vi "Main.vi"() -> ()   [LabVIEW 2021]
doc: "This software acquires data from an NI DAQ Device, displays it, and performs analysis of the data."
uses:
  controls/File Type.ctl
  controls/Data.ctl
  controls/Configuration Settings.ctl
  controls/State.ctl
panel:
  in  "Open File Location?":bool
  in  "File Type":T1
  out "Data":dbl[][](graph)
  out "Actual Sample Rate (Hz)":dbl
  in  "Copy Graph Data":bool
  in  "Copy Graph Image":bool
  in  "Reset Settings":bool
  in  "Clear Graph":bool
  in  "Read Data File":bool
  in  "Save to File":bool
  in  "Analyse Data":bool
  in  "Acquire Data":bool
  in  "Configure Data":bool
  out "Current State":string
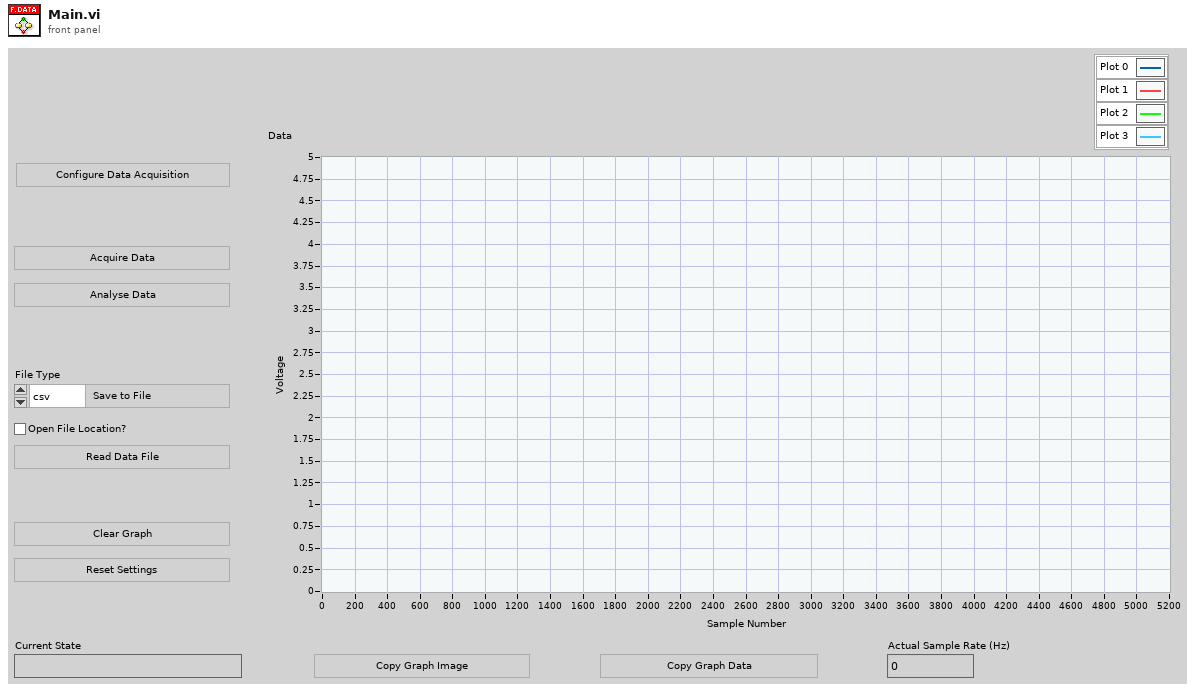
[diagram p1: front panel]
types:
  T1 = typedef "File Type.ctl" = enum16{"csv", "txt", "tdms"}
  T2 = typedef "State.ctl" = enum16{"Initialise", "Update User Interface", "Wait for Event", "Configure Data", "Acquire Data", "Reset Config Data", "Clear Data", "Analyse Data", "Save Data", "Open Data", "Error", "Stop"}
  T3 = typedef "Data.ctl" = cluster{"Configuration Settings":T4, "Data":dbl[][], "Actual Sample Rate (Hz)":dbl}
  T4 = typedef "Configuration Settings.ctl" = cluster{"Number of Samples":i32, "Desired Sample Rate (Hz)":dbl, "Minimum Value":dbl, "Maximum Value":dbl, "Physical Channels":tag}
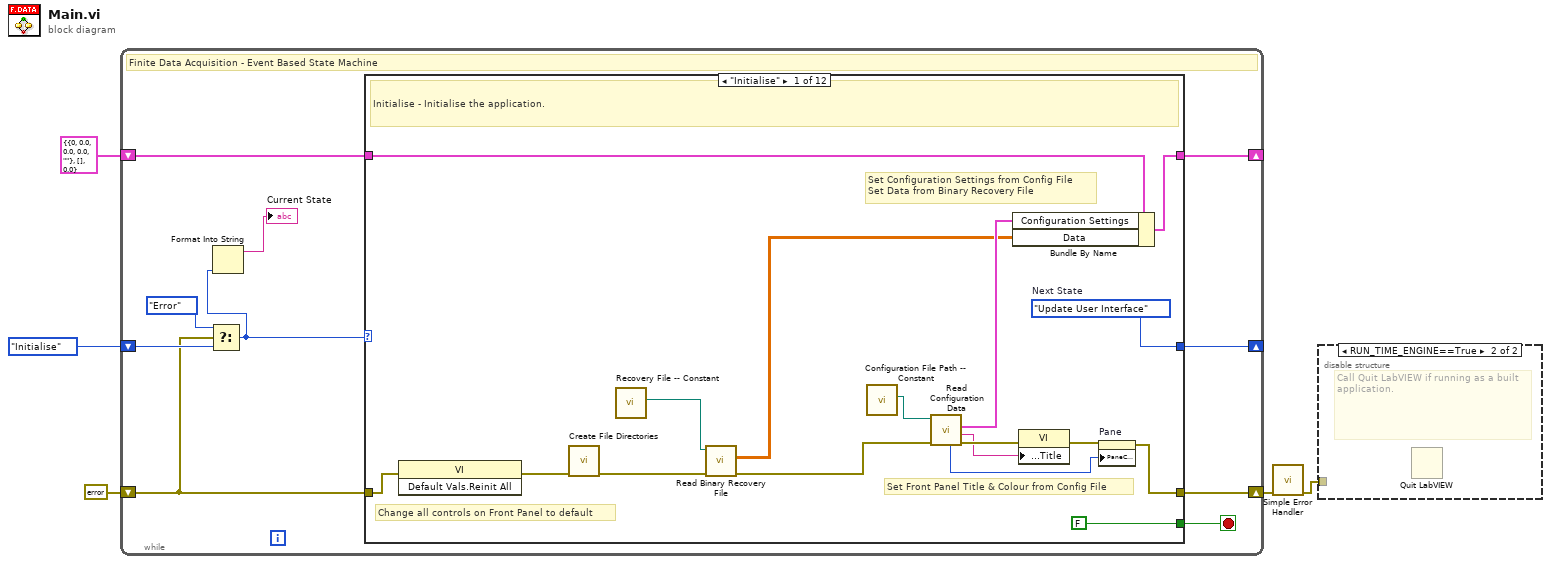
[diagram p0: block diagram]
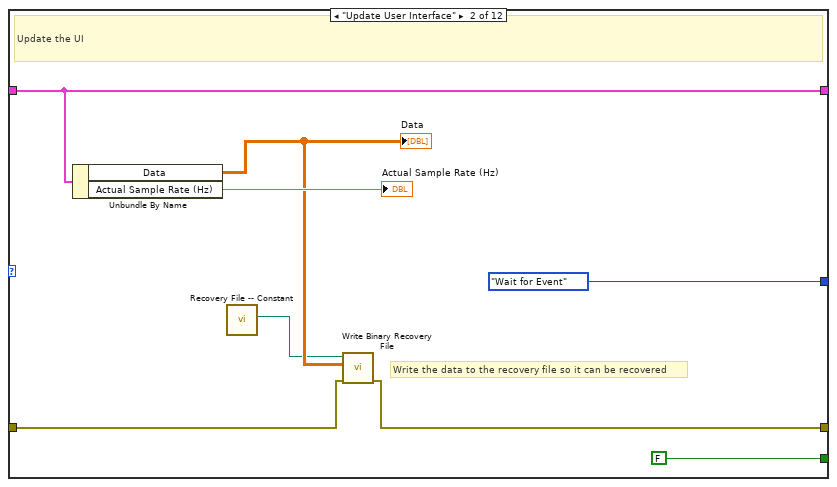
[diagram p3: hidden frame]
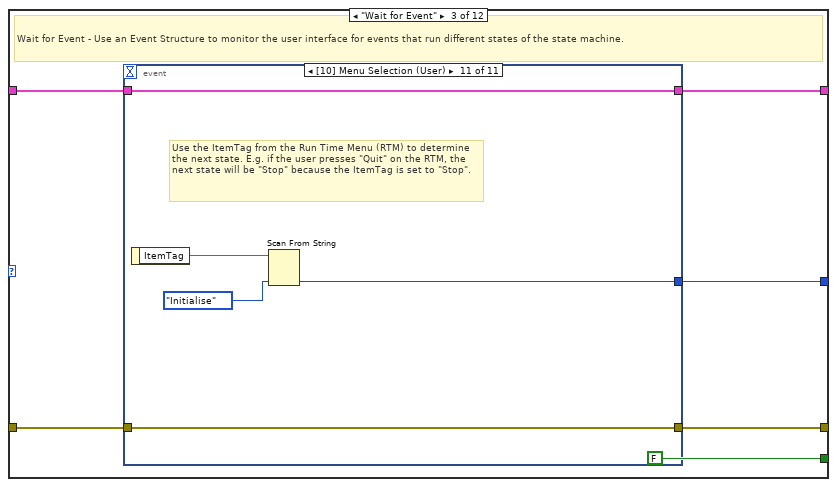
[diagram p4: hidden frame]
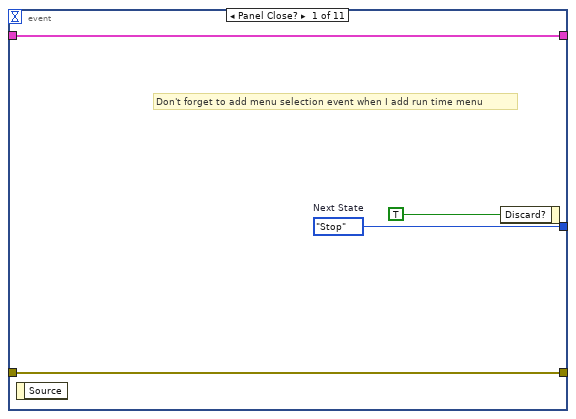
[diagram p5: hidden frame]
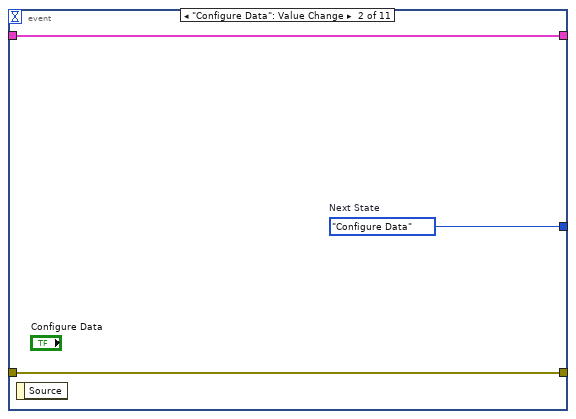
[diagram p6: hidden frame]
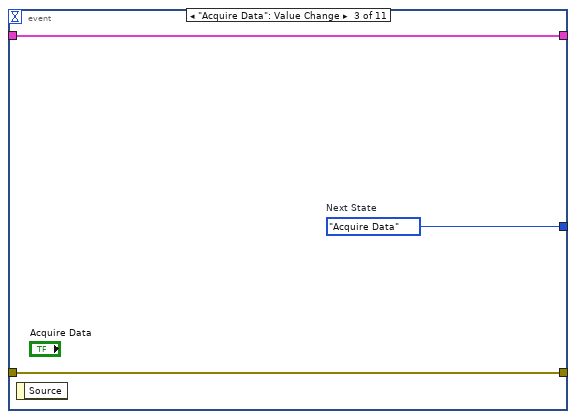
[diagram p7: hidden frame]
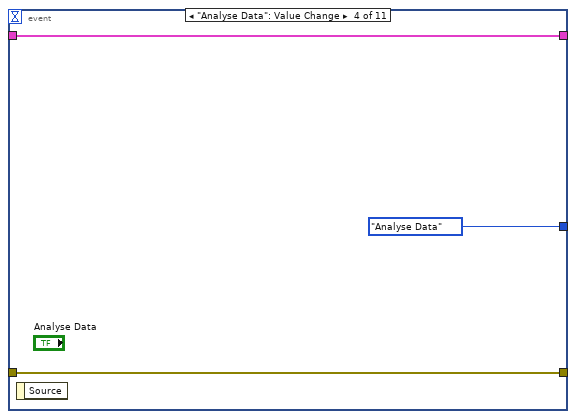
[diagram p8: hidden frame]
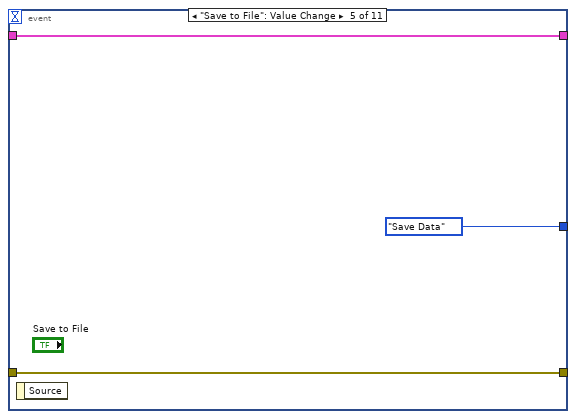
[diagram p9: hidden frame]
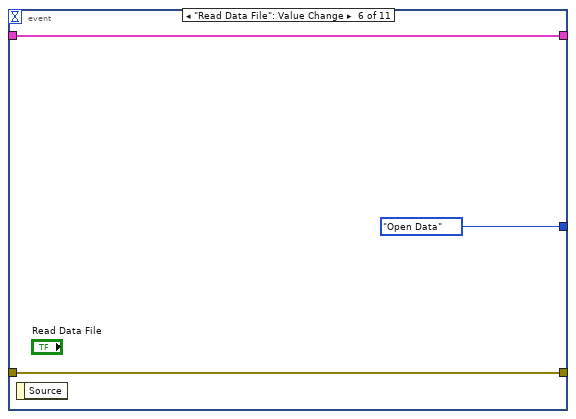
[diagram p10: hidden frame]
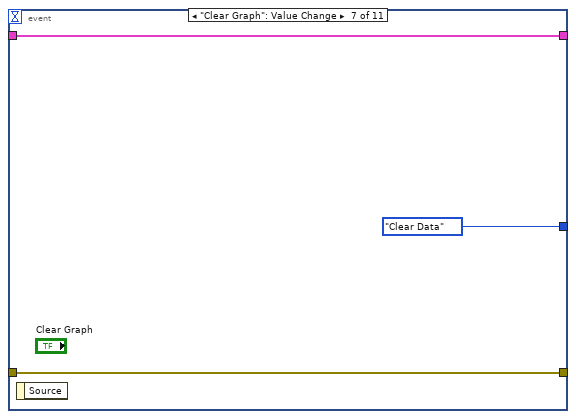
[diagram p11: hidden frame]
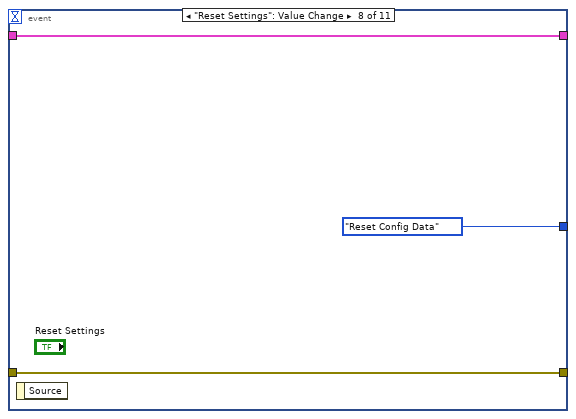
[diagram p12: hidden frame]
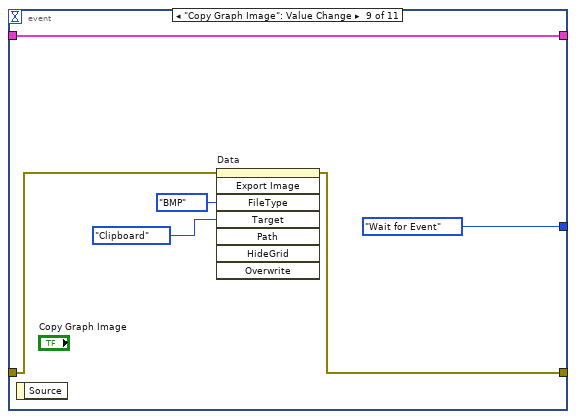
[diagram p13: hidden frame]
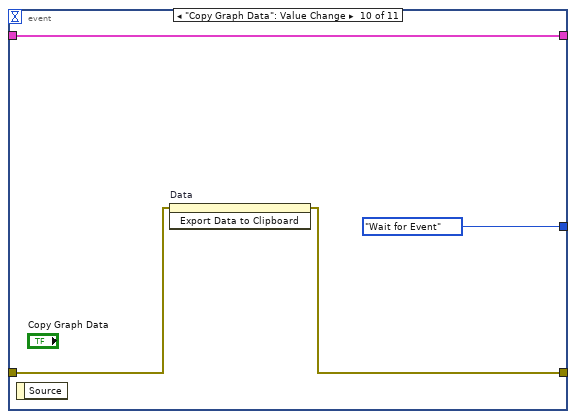
[diagram p14: hidden frame]
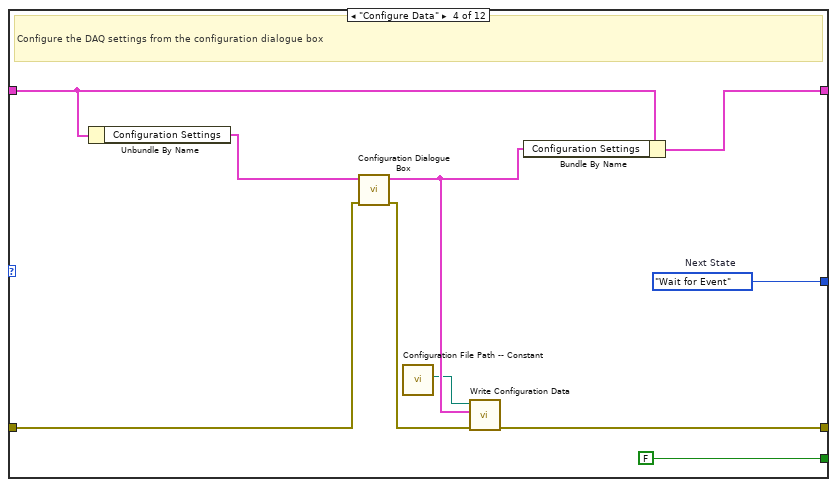
[diagram p15: hidden frame]
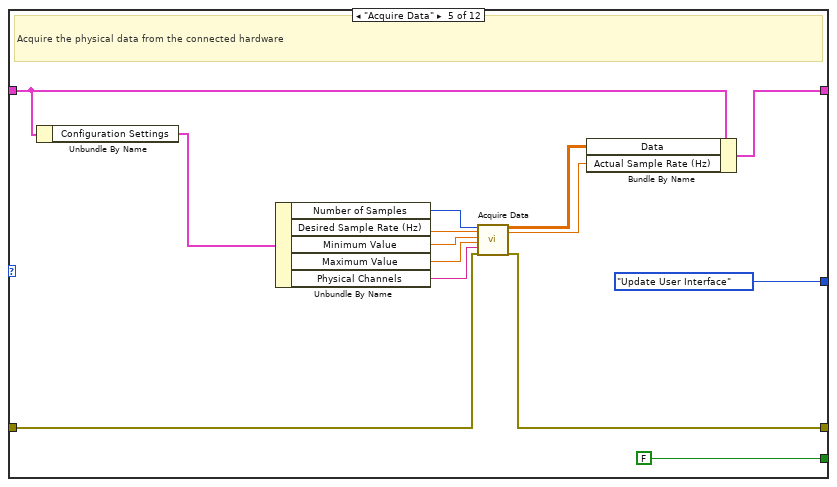
[diagram p16: hidden frame]
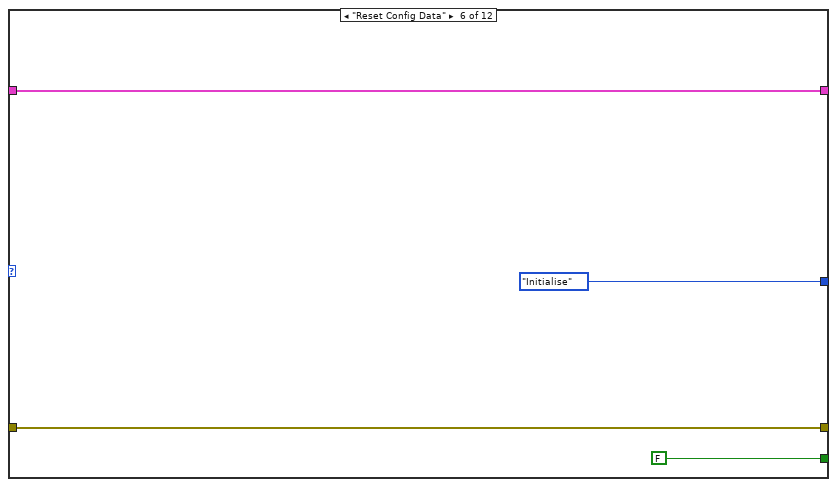
[diagram p17: hidden frame]
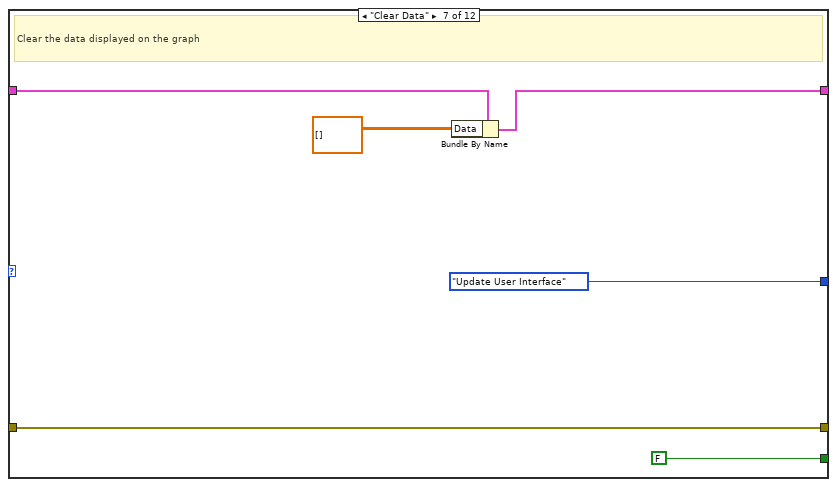
[diagram p18: hidden frame]
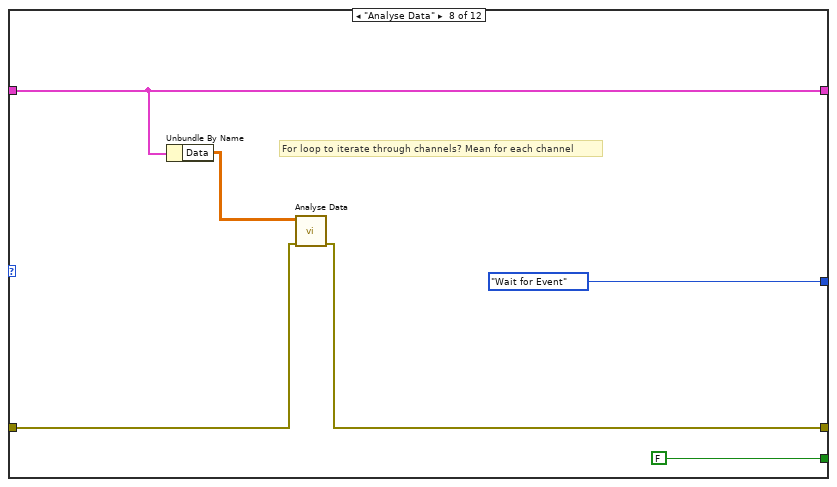
[diagram p19: hidden frame]
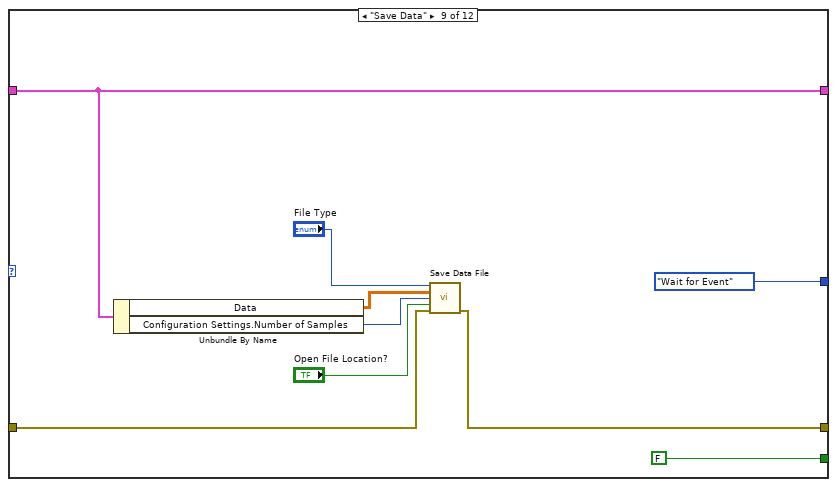
[diagram p20: hidden frame]
diagram:
  n1 = while {
    shift-right: [w15] -> _
    shift-left: State."Initialise" ("States") -> [w11]
    shift-right: [w13] -> _
    shift-left: T3 {"Configuration Settings"={"Number of Samples"=0, "Desired Sample Rate (Hz)"=0.0, "Minimum Value"=0.0, "Maximum Value"=0.0, "Physical Channels"=""}, "Data"=[], "Actual Sample Rate (Hz)"=0.0} ("Data") -> [w14]
    shift-right: [w12] -> w3
    shift-left: errorcluster {"status"=FALSE, "code"=0, "source"=""} ("error constant") -> [w9]
    stop <- w6 stop-if-true
    # "Finite Data Acquisition - Event Based State Machine"
    n2 = Select(t=State."Error", s=w9, f=w11) -> (s? t:f=w8:T2)
    n3 = Format Into String(w8) -> (resulting string=→"Current State":string)  [unwired: 3 in, 1 out]
    n4 = case shown="\"Initialise\"" w8 {
      tunnel: [w32 State."Wait for Event" ("(Value Not Used)") w46 w96 State."Update User Interface" State."Initialise" State."Update User Interface" State."Wait for Event" State."Wait for Event" w137 State."Stop" _] -> w15
      tunnel: [FALSE ("Stop Loop?") FALSE ("Stop Loop?") FALSE ("Stop Loop?") FALSE ("Stop Loop?") FALSE ("Stop Loop?") FALSE ("Stop Loop?") FALSE ("Stop Loop?") FALSE ("Stop Loop?") FALSE ("Stop Loop?") FALSE ("Stop Loop?") _ TRUE ("Stop Loop?")] -> w6
      tunnel: w14 -> [w30 w38 w44 w92 w100 w114 w117 w124 w133 w139 w191 w194]
      tunnel: [w29 w38 w43 w91 w99 w114 w116 w124 w133 w138 w191 w194] -> w13
      tunnel: w9 -> [w21 w34 w42 w93 w102 w113 w120 w122 w131 w143 w188 w193]
      tunnel: [w22 w33 w41 w87 w101 w113 w120 w121 w130 w136 errorcluster {"status"=FALSE, "code"=0, "source"=""} ("error in (no error)") w193] -> w12
      frame "Initialise" {
        w32 = State."Update User Interface"  # Next State
        # "Change all controls on Front Panel to default"
        # "Set Configuration Settings from Config File\nSet Data from Binary Recovery File"
        # "Set Front Panel Title & Colour from Config File"
        # "Initialise - Initialise the application."
        n5 = invoke class="VI" method="Default Vals.Reinit All"(error in=w21) -> (error out=w16:errorcluster)  [unwired: 2 in, 2 out]
        n6 = call "Create File Directories.vi"("error in"=w16) -> ("error out"=w20:errorcluster)  [unwired: 10 in]
        n7 = call "Recovery File -- Constant.vi"() -> ("Recovery File Path"=w19:path)  [unwired: 11 in]
        n8 = call "Read Binary Recovery File.vi"("error in"=w20, "File Path"=w19) -> ("error out"=w17:errorcluster, "Data Out"=w18:dbl[][])  [unwired: 8 in]
        n9 = call "Configuration File Path -- Constant.vi"() -> ("Configuration File Path"=w27:path)  [unwired: 11 in]
        n10 = call "Read Configuration Data.vi"("error in"=w17, "File Path"=w27) -> ("error out"=w26:errorcluster, "VI Title"=w25:string, "Configuration Settings"=w28:T4, "Panel Colour"=w24:u32)  [unwired: 6 in]
        n11 = Bundle By Name(cluster=w30, "Configuration Settings"=w28, "Data"=w18) -> (w29:T3)
        n12 = property class="VI"(error in=w26, "Front Panel.Title"=w25) -> (error out=w23:errorcluster)  [unwired: 1 in, 1 out]
        n13 = property on="Pane" class="Pane"(error in=w23, "PaneColor"=w24) -> (error out=w22:errorcluster)  [unwired: 1 in, 1 out]
      }
      frame "Update User Interface" {
        # "Write the data to the recovery file so it can be recovered"
        # "Update the UI"
        n14 = Unbundle By Name(w38) -> ("Data"=w36:dbl[][], "Actual Sample Rate (Hz)"=→"Actual Sample Rate (Hz)":dbl)
        "Data" <- w36
        n15 = call "Recovery File -- Constant.vi"() -> ("Recovery File Path"=w35:path)  [unwired: 11 in]
        n16 = call "Write Binary Recovery File.vi"("error in"=w34, "Data In"=w36, "File Path"=w35) -> ("error out"=w33:errorcluster)  [unwired: 8 in]
      }
      frame "Wait for Event" {
        # "Wait for Event - Use an Event Structure to monitor the user interface for events that run different states of the state machine."
        n17 = event shown="[10] Menu Selection (User)" {
          selector: _ -> [_ _ _ _ _ _ _ _ _ _ _]
          dyn-events: _ -> [_ _ _ _ _ _ _ _ _ _ _]
          timeout: _ -> [_ _ _ _ _ _ _ _ _ _ _]
          tunnel: [w50 w53 w56 State."Analyse Data" ("Next State") State."Save Data" ("Next State") State."Open Data" ("Next State") State."Clear Data" ("Next State") State."Reset Config Data" ("Next State") State."Wait for Event" ("Next State") State."Wait for Event" ("Next State") w82] -> w46
          tunnel: w44 -> [w49 w51 w54 w59 w62 w65 w68 w71 w77 w81 w86]
          tunnel: [w49 w51 w54 w59 w62 w65 w68 w71 w77 w81 w86] -> w43
          tunnel: w42 -> [w48 w52 w55 w58 w61 w64 w67 w70 w73 w79 w85]
          tunnel: [w48 w52 w55 w58 w61 w64 w67 w70 w72 w78 w85] -> w41
          event Panel Close? {
            w50 = State."Stop"  # Next State
            # "Don't forget to add menu selection event when I add run time menu"
            n18 = event-data() -> ()  [unwired: 1 in, 1 out]
            n19 = event-data("Discard?"=TRUE) -> ()  [unwired: 1 in, 1 out]
          }
          event "Configure Data": Value Change {
            w53 = State."Configure Data"  # Next State
            n20 = event-data() -> ()  [unwired: 1 in, 1 out]
          }
          event "Acquire Data": Value Change {
            w56 = State."Acquire Data"  # Next State
            n21 = event-data() -> ()  [unwired: 1 in, 1 out]
          }
          event "Analyse Data": Value Change {
            n22 = event-data() -> ()  [unwired: 1 in, 1 out]
          }
          event "Save to File": Value Change {
            n23 = event-data() -> ()  [unwired: 1 in, 1 out]
          }
          event "Read Data File": Value Change {
            n24 = event-data() -> ()  [unwired: 1 in, 1 out]
          }
          event "Clear Graph": Value Change {
            n25 = event-data() -> ()  [unwired: 1 in, 1 out]
          }
          event "Reset Settings": Value Change {
            n26 = event-data() -> ()  [unwired: 1 in, 1 out]
          }
          event "Copy Graph Image": Value Change {
            n27 = event-data() -> ()  [unwired: 1 in, 1 out]
            n28 = invoke on="Data" class="WFGraph (strict)" method="Export Image"(error in=w73, "FileType"=enum32{"BMP", "EPS", "EMF", "PICT"}."BMP" ("File Type"), "Target"=enum32{"File", "Clipboard"}."Clipboard") -> (error out=w72:errorcluster)  [unwired: 5 in, 7 out]
          }
          event "Copy Graph Data": Value Change {
            n29 = event-data() -> ()  [unwired: 1 in, 1 out]
            n30 = invoke on="Data" class="WFGraph (strict)" method="Export Data to Clipboard"(error in=w79) -> (error out=w78:errorcluster)  [unwired: 2 in, 2 out]
          }
          event Menu Selection (User) {
            # "Use the ItemTag from the Run Time Menu (RTM) to determine the next state. E.g. if the user presses \"Quit\" on the RTM, the next state will be \"Stop\" because the ItemTag is set to \"Stop\"."
            n31 = event-data() -> ("ItemTag"=w84:string)  [unwired: 1 in]
            n32 = Scan From String "Scan From String"(input string=w84, default 1=State."Initialise" ("States")) -> (output 1=w82:T2)  [unwired: 3 in, 3 out]
          }
        }
      }
      frame "Configure Data" {
        w96 = State."Wait for Event"  # Next State
        # "Configure the DAQ settings from the configuration dialogue box"
        n33 = Unbundle By Name(w92) -> ("Configuration Settings"=w94:T4)
        n34 = call "Configuration Dialogue Box.vi"("error in"=w93, "Configuration Settings In"=w94) -> ("error out"=w88:errorcluster, "Configuration Settings Out"=w90:T4)  [unwired: 8 in]
        n35 = call "Configuration File Path -- Constant.vi"() -> ("Configuration File Path"=w89:path)  [unwired: 11 in]
        n36 = call "Write Configuration Data.vi"("error in"=w88, "Configuration Settings"=w90, "File Path"=w89) -> ("error out"=w87:errorcluster)  [unwired: 8 in]
        n37 = Bundle By Name(cluster=w92, "Configuration Settings"=w90) -> (w91:T3)
      }
      frame "Acquire Data" {
        # "Acquire the physical data from the connected hardware"
        n38 = Unbundle By Name(w100) -> ("Configuration Settings"=w109:T4)
        n39 = Unbundle By Name(w109) -> ("Number of Samples"=w107:i32, "Desired Sample Rate (Hz)"=w106:dbl, "Minimum Value"=w105:dbl, "Maximum Value"=w104:dbl, "Physical Channels"=w103:tag)
        n40 = call "Acquire Data.vi"("Number of Samples"=w107, "Desired Sample Rate (Hz)"=w106, "Minimum Value"=w105, "Maximum Value"=w104, "Physical Channels"=w103, "error in"=w102) -> ("Data Out"=w98:dbl[][], "Actual Sample Rate (Hz)"=w97:dbl, "error out"=w101:errorcluster)  [unwired: 11 in]
        n41 = Bundle By Name(cluster=w100, "Data"=w98, "Actual Sample Rate (Hz)"=w97) -> (w99:T3)
      }
      frame "Reset Config Data" {
      }
      frame "Clear Data" {
        # "Clear the data displayed on the graph"
        n42 = Bundle By Name(cluster=w117, "Data"=dbl[][] []) -> (w116:T3)
      }
      frame "Analyse Data" {
        # "For loop to iterate through channels? Mean for each channel"
        n43 = Unbundle By Name(w124) -> ("Data"=w123:dbl[][])
        n44 = call "Analyse Data.vi"("error in"=w122, "Data"=w123) -> ("error out"=w121:errorcluster)  [unwired: 9 in]
      }
      frame "Save Data" {
        n45 = Unbundle By Name(w133) -> ("Data"=w132:dbl[][], "Configuration Settings.Number of Samples"=w129:i32)
        n46 = call "Save Data File.vi"("File Type"="File Type", "Data"=w132, "Number of Samples"=w129, "Open File Location?"="Open File Location?", "error in"=w131) -> ("error out"=w130:errorcluster)  [unwired: 10 in]
      }
      frame "Open Data" {
        n47 = call "Data File Directory -- Constant.vi"() -> ("Data File Directory"=w147:path)  [unwired: 11 in]
        n48 = call "File Dialog"("start path"=w147, "prompt"="Select a data\nfile to open", "default name"="*.txt;*.csv;*.tdms", "error in"=w143, "pattern label"="Data Files Finite DAQ") -> ("selected path"=w141:path, "cancelled"=w140:bool, "error out"=w142:errorcluster)  [unwired: 7 in, 1 out]
        n49 = case shown="False" w140 {
          tunnel: [w152 State."Wait for Event"] -> w137
          tunnel: w142 -> [w157 w186]
          tunnel: w141 -> [w155 _]
          tunnel: [w149 w185] -> w136
          tunnel: w139 -> [w151 w183]
          tunnel: [w150 w183] -> w138
          frame False {
            # "The user selected a file"
            n50 = call <vilib>:"Get File Extension.vi"("error in (no error)"=w157, "file"=w155) -> ("error out"=w153:errorcluster, "lowercase file extension"=w156:string, "dup file"=w154:path)  [unwired: 5 in, 2 out]
            n51 = case shown="\"tdms\"" w156 {
              tunnel: w154 -> [_ w167 w172 w181]
              tunnel: w153 -> [w158 w166 w174 w182]
              tunnel: [State."Wait for Event" State."Update User Interface" State."Update User Interface" State."Update User Interface"] -> w152
              tunnel: w151 -> [w159 w164 w171 w180]
              tunnel: [w159 w163 w170 w179] -> w150
              tunnel: [w158 w165 w173 w176] -> w149
              frame Default {
                n52 = One Button Dialog(message="File type not supported") -> ()  [unwired: 1 in, 1 out]
              }
              frame "tdms" {
                n53 = call "Read TDMS File.vi"("error in"=w166, "File Path"=w167) -> ("error out"=w165:errorcluster, "Data Out"=w162:dbl[][])  [unwired: 8 in]
                n54 = Bundle By Name(cluster=w164, "Data"=w162) -> (w163:T3)
              }
              frame "csv" {
                n55 = call "Read CSV File.vi"("error in"=w174, "File Path"=w172) -> ("error out"=w173:errorcluster, "Data Out"=w169:dbl[][])  [unwired: 8 in]
                n56 = Bundle By Name(cluster=w171, "Data"=w169) -> (w170:T3)
              }
              frame "txt" {
                n57 = call "Read Text File.vi"("error in"=w182, "File Path"=w181) -> ("error out"=w176:errorcluster, "Data Out"=w178:dbl[][])  [unwired: 8 in]
                n58 = Bundle By Name(cluster=w180, "Data"=w178) -> (w179:T3)
              }
            }
          }
          frame True {
            # "The user cancelled the file dialog"
            n59 = call <vilib>:"Clear Errors.vi"("error in (no error)"=w186, "specific error code to clear (0: all)"=43) -> ("error out"=w185:errorcluster)  [unwired: 4 in, 1 out]
          }
        }
      }
      frame "Error" {
        n60 = call <vilib>:"Simple Error Handler.vi"("error in (no error)"=w188) -> ()  [unwired: 4 in, 5 out]
      }
      frame "Stop" {
        # "Stop the application"
      }
    }
  }
  n61 = call <vilib>:"Simple Error Handler.vi"("error in (no error)"=w3) -> ("error out"=w2:errorcluster)  [unwired: 4 in, 4 out]
  n62 = disable-structure shown="RUN_TIME_ENGINE==True" {
    disable-tunnel: w2 -> [_ _]
    frame condition #0 (active) {
    }
    frame condition #1 {
      # "Call Quit LabVIEW if running as a built application."
      n63 = Quit LabVIEW() -> ()  [unwired: 1 in]
    }
  }
